vi "Parse Address.vi"(7 "SPI_Mode":T1, 8 "error in (no error)":errorcluster, 11 "Addr in":string) -> (0 "error out":errorcluster, 3 "Addr out":u16)   [LabVIEW 2018, in "Config_Read_SPI.lvclass"]
uses:
  Config_Read_SPI.lvclass
  SPI_Mode.ctl
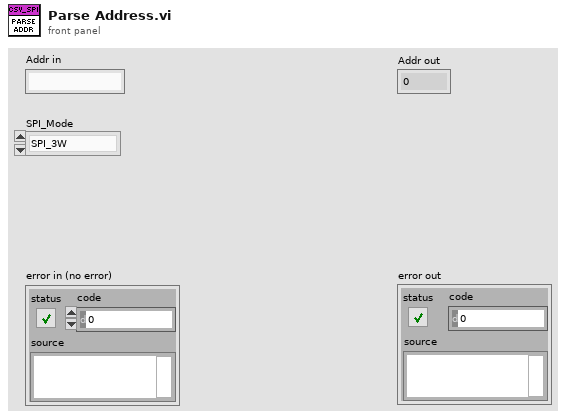
[diagram p1: front panel]
types:
  T1 = typedef "Config_Read_SPI.lvclass/SPI_Mode.ctl" = enum16{"SPI_3W", "SPI_4W"}
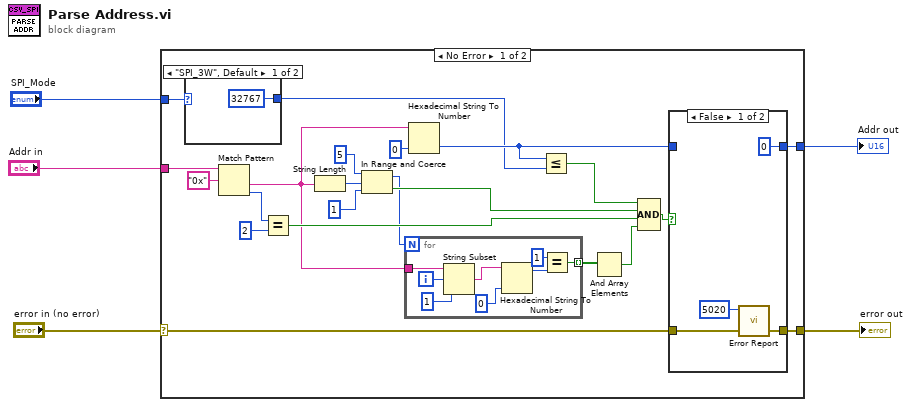
[diagram p0: block diagram]
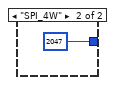
[diagram p2: hidden frame]
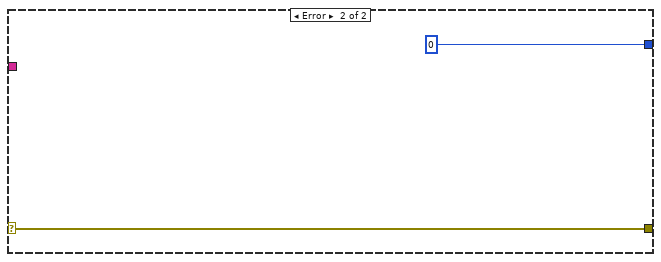
[diagram p4: hidden frame]
diagram:
  n1 = case shown="No Error" "error in (no error)" {
    selector: "error in (no error)" -> [w20 w45]
    tunnel: "Addr in" -> [w27 _]
    tunnel: [w19 w45] -> w3
    tunnel: [w18 u16 0] -> w2
    tunnel: "SPI_Mode" -> [w7 _]
    frame No Error {
      n2 = case shown="\"SPI_3W\", Default" w7 {
        tunnel: [u16 32767 ("y") u16 2047 ("y")] -> w6
        frame "SPI_3W", Default {
        }
        frame "SPI_4W" {
        }
      }
      n3 = Match Pattern(string=w27, regular expression="0x") -> (after substring=w12:string, offset past match=w25:i32)  [unwired: 1 in, 2 out]
      n4 = Equal?(x=w25, y=2) -> (x = y?=w22:bool)
      n5 = String Length(string=w12) -> (length=w17:i32)
      n6 = In Range and Coerce(upper limit=5, x=w17, lower limit=1 ("upper limit")) -> (coerced(x)=w13:i32, In Range?=w14:bool)
      n7 = for {
        N: w13 -> [_]
        tunnel: w12 -> [w37]
        tunnel: [w30] -> w11 mode=indexing
        i -> [w36]
        n8 = String Subset(string=w37, offset (0)=w36, length (rest)=1 ("length (rest)")) -> (substring=w34:string)
        n9 = Hexadecimal String To Number(string=w34, default (0uL)=u16 0 ("Addr out")) -> (offset past number=w32:i32)  [unwired: 1 in, 1 out]
        n10 = Equal?(x=1, y=w32) -> (x = y?=w30:bool)
      }
      n11 = Hexadecimal String To Number(string=w12, default (0uL)=u16 0 ("Addr out")) -> (number=w9:u16)  [unwired: 1 in, 1 out]
      n12 = Less Or Equal?(x=w9, y=w6) -> (x <= y?=w8:bool)
      n13 = And Array Elements(Boolean array=w11) -> (logical AND=w10:bool)
      n14 = Compound Arithmetic op=AND(w8, w14, w22, w10) -> (w21:bool)
      n15 = case shown="False" w21 {
        tunnel: w20 -> [w38 w43]
        tunnel: w9 -> [_ w42]
        tunnel: [w40 w43] -> w19
        tunnel: [u16 0 w42] -> w18
        frame False {
          n16 = call "Error Report.vi"("error in (no error)"=w38, "Error Code"=i16 5020) -> ("error out"=w40:errorcluster)  [unwired: 9 in]
        }
        frame True {
        }
      }
    }
    frame Error {
    }
  }
  "error out" <- w3
  "Addr out" <- w2
